vi "Calculate Driving Direction.vi"(8 "error in (no error)":errorcluster, 10 "obstacle angles (rad)":dbl[](array[numeric]), 11 "obstacle distances (m)":dbl[](array[numeric])) -> (0 "error out":errorcluster, 3 "steering frame velocity":dbl[](array[numeric]), 9 "x.or.y?":bool)   [LabVIEW 2015]
doc: "Calculates the velocity vector of the robot required to avoid obstacles, based on the scanned data."
uses:
  <vilib>/robotics/Obstacle Avoidance/Simple Vector Field Histogram/Panic Range.ctl
  <vilib>/Utility/AngleManip/Degrees to Radians (Scalar DBL).vi
  <vilib>/robotics/Obstacle Avoidance/Simple Vector Field Histogram/NI_Robotics_Simple Vector Field Histogram.lvlib
  <vilib>/Utility/AngleManip/NI_AngleManipulation.lvlib
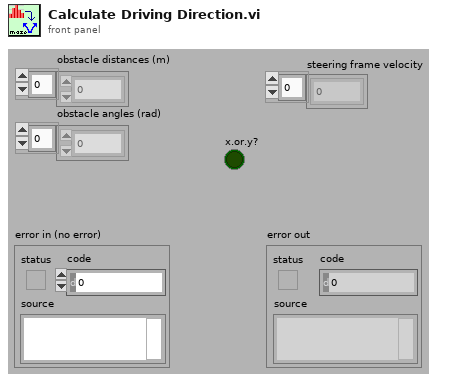
[diagram p1: front panel]
types:
  T1 = typedef "NI_Robotics_Simple Vector Field Histogram.lvlib/Panic Range.ctl" = cluster{"panic threshold distance (0)":dbl, "panic threshold angle (0)":dbl}
  T2 = typedef "NI_Robotics_Simple Vector Field Histogram.lvlib/Obstacle Description.ctl" = cluster{"angle to obstacle":dbl, "distance to obstacle":dbl}
  T3 = typedef "NI_Robotics_Simple Vector Field Histogram.lvlib/Gap Description.ctl" = cluster{"angle to gap":dbl, "size of gap":dbl}
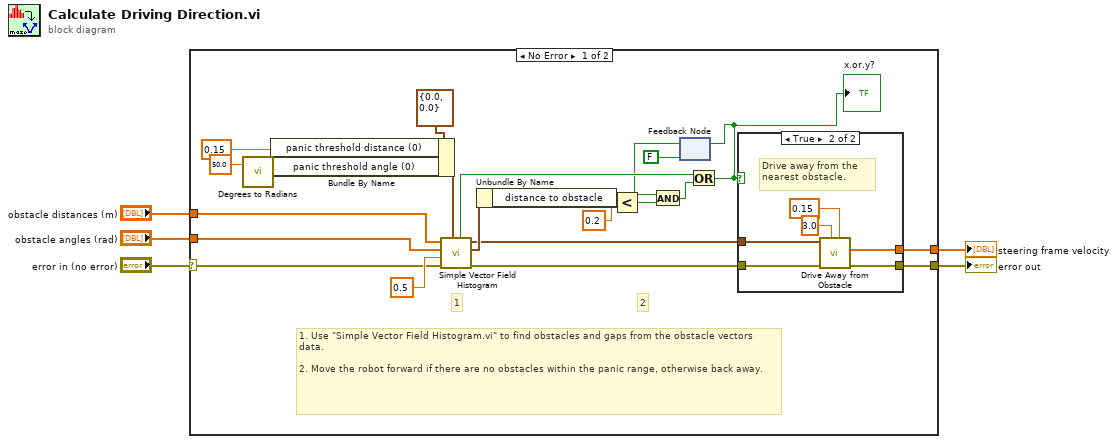
[diagram p0: block diagram]
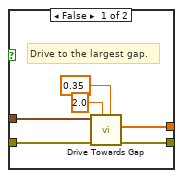
[diagram p2: hidden frame]
diagram:
  n1 = case shown="No Error" "error in (no error)" {
    selector: "error in (no error)" -> [w11 w40]
    tunnel: [w12 w40] -> w5
    tunnel: "obstacle distances (m)" -> [w10 _]
    tunnel: "obstacle angles (rad)" -> [w9 _]
    tunnel: [w8 _] -> w1
    frame No Error {
      # "2"
      # "1"
      # "1. Use \"Simple Vector Field Histogram.vi\" to find obstacles and gaps from the obstacle vectors data.\n\n2. Move the robot forward if there are no obstacles within the panic range, otherwise back away."
      n2 = call-poly <vilib>:"Degrees to Radians.vi"("angle (deg)"=50.0 ("panic threshold angle (rad)")) -> ("angle (rad)"=w27:dbl)  [unwired: 2 in]
      n3 = Bundle By Name(cluster=T1 {"panic threshold distance (0)"=0.0, "panic threshold angle (0)"=0.0} ("panic range"), "panic threshold distance (0)"=0.15 ("panic threshold distance (m)"), "panic threshold angle (0)"=w27) -> (w16:T1)
      n4 = call <vilib>:"Simple Vector Field Histogram.vi"("panic range"=w16, "error in (no error)"=w11, "distance threshold"=0.5 ("distance threshold (m)"), "direction angles"=w9, "distances"=w10) -> ("error out"=w13:errorcluster, "nearest obstacle"=w18:T2, "largest gap"=w7:T3, "obstacle within panic range"=w23:bool)  [unwired: 2 in, 1 out]
      n5 = Unbundle By Name(w18) -> ("distance to obstacle"=w19:dbl)
      n6 = Less?(x=w19, y=0.2) -> (x < y?=w21:bool)
      n7 = feedback #1(FALSE ("obstacle within panic range")) -> (w22:bool)
      n8 = And(x=w22, y=w21) -> (x .and. y?=w24:bool)
      n9 = Or(x=w23, y=w24) -> (x .or. y?=w6:bool)
      "x.or.y?" <- w6
      n10 = feedback-in #1(w6) -> ()
      n11 = case shown="True" w6 {
        tunnel: w7 -> [w32 w37]
        tunnel: w13 -> [w33 w39]
        tunnel: [w31 w38] -> w12
        tunnel: [w30 w36] -> w8
        frame False {
          # "Drive to the largest gap."
          n12 = call "Drive Towards Gap.vi"("max forward velocity (m/s)"=0.35, "max angular velocity (rad/s)"=2.0, "error in (no error)"=w33, "gap"=w32) -> ("error out"=w31:errorcluster, "steering frame velocity"=w30:dbl[])  [unwired: 6 in]
        }
        frame True {
          # "Drive away from the nearest obstacle."
          n13 = call "Drive Away from Obstacle.vi"("max reverse velocity (m/s)"=0.15, "max angular velocity (rad/s)"=3.0, "error in (no error)"=w39, "gap"=w37) -> ("error out"=w38:errorcluster, "steering frame velocity"=w36:dbl[])  [unwired: 6 in]
        }
      }
    }
    frame Error {
    }
  }
  "error out" <- w5
  "steering frame velocity" <- w1
